vi "set_red_state.vi"(0 "字符串":string, 7 "red":T1) -> (4 "set":T1)   [LabVIEW 2012]
uses:
  <vilib>/Embedded/WSN/Error codes.ctl
  <vilib>/LabVIEW Targets/Embedded/WSN/RadioMessages.xnode
panel:
  out "index":i32
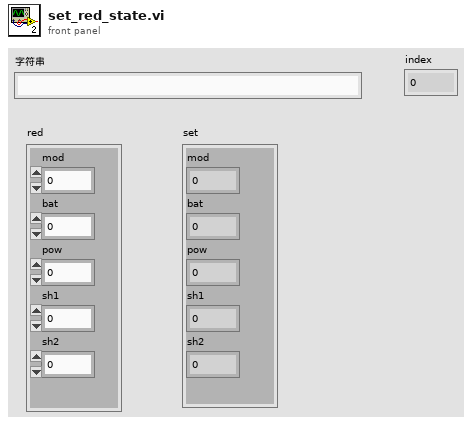
[diagram p1: front panel]
types:
  T1 = cluster{"mod":i32, "bat":i32, "pow":i32, "sh1":i32, "sh2":i32}
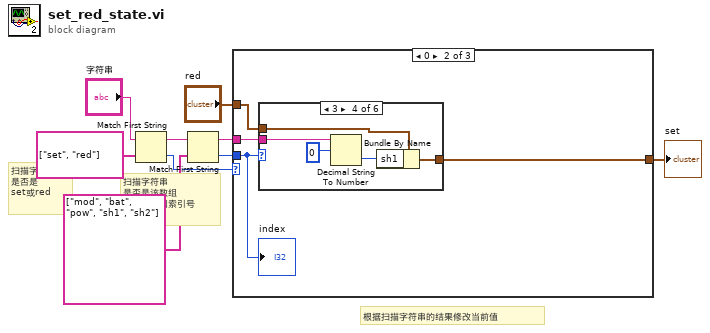
[diagram p0: block diagram]
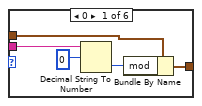
[diagram p3: hidden frame]
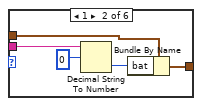
[diagram p4: hidden frame]
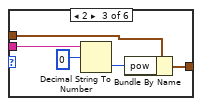
[diagram p5: hidden frame]
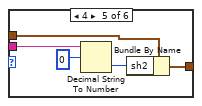
[diagram p6: hidden frame]
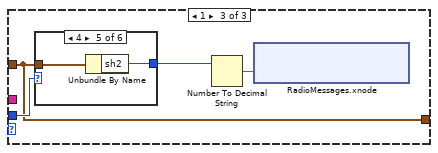
[diagram p8: hidden frame]
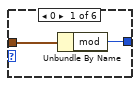
[diagram p9: hidden frame]
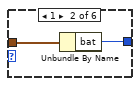
[diagram p10: hidden frame]
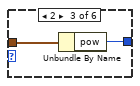
[diagram p11: hidden frame]
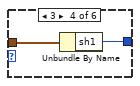
[diagram p12: hidden frame]
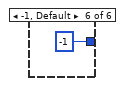
[diagram p13: hidden frame]
diagram:
  # "根据扫描字符串的结果修改当前值"
  # "扫描字符串\n是否是该数组\n里的，返回索引号"
  # "扫描字符串\n是否是\nset或red"
  n1 = Match First String(2:string[] ["set", "red"] ("字符串数组"), 3:"字符串") -> (0:w4:i32, 1:w5:string)
  n2 = Match First String(2:string[] ["mod", "bat", "pow", "sh1", "sh2"] ("字符串数组"), 3:w5) -> (0:w9:i32, 1:w8:string)
  n3 = case shown="0" w4 {
    tunnel: w9 -> [_ w14 w44]
    tunnel: w8 -> [_ w13 _]
    tunnel: "red" -> [w10 w11 w41]
    tunnel: [w10 w12 w41] -> w1
    frame -1, Default {
    }
    frame 0 {
      n4 = case shown="3" w14 {
        tunnel: w13 -> [w18 w22 w29 w33 w38 _]
        tunnel: [w15 w20 w25 w30 w36 w40] -> w12
        tunnel: w11 -> [w16 w21 w26 w31 w35 w40]
        frame 0 {
          n5 = Decimal String To Number(string=w18, offset=0 ("偏移量")) -> (number=w17:i32)  [unwired: 1 in, 1 out]
          n6 = Bundle By Name(cluster=w16, "mod"=w17) -> (w15:T1)
        }
        frame 1 {
          n7 = Decimal String To Number(string=w22, offset=0 ("偏移量")) -> (number=w23:i32)  [unwired: 1 in, 1 out]
          n8 = Bundle By Name(cluster=w21, "bat"=w23) -> (w20:T1)
        }
        frame 2 {
          n9 = Decimal String To Number(string=w29, offset=0 ("偏移量")) -> (number=w27:i32)  [unwired: 1 in, 1 out]
          n10 = Bundle By Name(cluster=w26, "pow"=w27) -> (w25:T1)
        }
        frame 3 {
          n11 = Decimal String To Number(string=w33, offset=0 ("偏移量")) -> (number=w32:i32)  [unwired: 1 in, 1 out]
          n12 = Bundle By Name(cluster=w31, "sh1"=w32) -> (w30:T1)
        }
        frame 4 {
          n13 = Decimal String To Number(string=w38, offset=0 ("偏移量")) -> (number=w37:i32)  [unwired: 1 in, 1 out]
          n14 = Bundle By Name(cluster=w35, "sh2"=w37) -> (w36:T1)
        }
        frame -1, Default {
        }
      }
      "index" <- w14
    }
    frame 1 {
      n15 = case shown="4" w44 {
        tunnel: [w50 w52 w54 w56 w58 -1] -> w43
        tunnel: w41 -> [w51 w53 w55 w57 w59 _]
        frame 0 {
          n16 = Unbundle By Name(w51) -> ("mod"=w50:i32)
        }
        frame 1 {
          n17 = Unbundle By Name(w53) -> ("bat"=w52:i32)
        }
        frame 2 {
          n18 = Unbundle By Name(w55) -> ("pow"=w54:i32)
        }
        frame 3 {
          n19 = Unbundle By Name(w57) -> ("sh1"=w56:i32)
        }
        frame 4 {
          n20 = Unbundle By Name(w59) -> ("sh2"=w58:i32)
        }
        frame -1, Default {
        }
      }
      n21 = Number To Decimal String(number=w43) -> (decimal integer string=w42:string)  [unwired: 1 in]
      n22 = xnode "RadioMessages.xnode"("sendUserMessage"=w42) -> ()  [unwired: 2 out]
    }
  }
  "set" <- w1
